vi "Hz to ms.vi"(4 "Hz input":dbl) -> (1 "ms output":dbl)   [LabVIEW 2020]
panel:
  in  "Tab Control":enum32{"Input", "Output"}(tab)
  # "Description: \nConverts hertz to milliseconds"
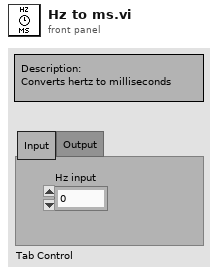
[diagram p1: front panel]
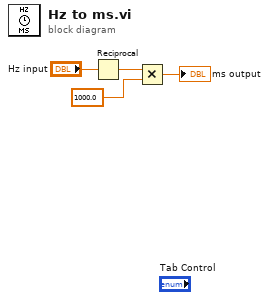
[diagram p0: block diagram]
diagram:
  n1 = Reciprocal(x="Hz input") -> (1/x=w4:dbl)
  n2 = Multiply(x=w4, y=1000.0) -> (x*y=→"ms output":dbl)
